vi "qmeter_calculation.vi"(1 "Range size":u16, 4 "Sample type":u16, 5 "Input voltage":dbl, 6 "stray capacitance":dbl, 7 "knob":dbl, 9 "phi":dbl, 10 "eta":dbl, 11 "trim":dbl) -> (2 "Cluster":cluster{"all rows":dbl[], "all rows":dbl[]})   [LabVIEW 2019]
uses:
  <vilib>/Utility/file.llb/Read Delimited Spreadsheet (DBL).vi
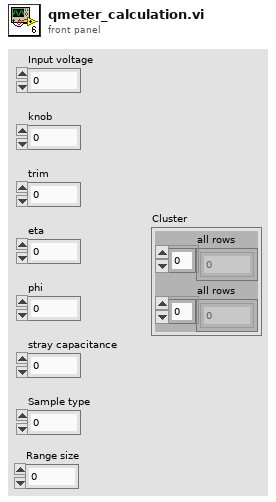
[diagram p1: front panel]
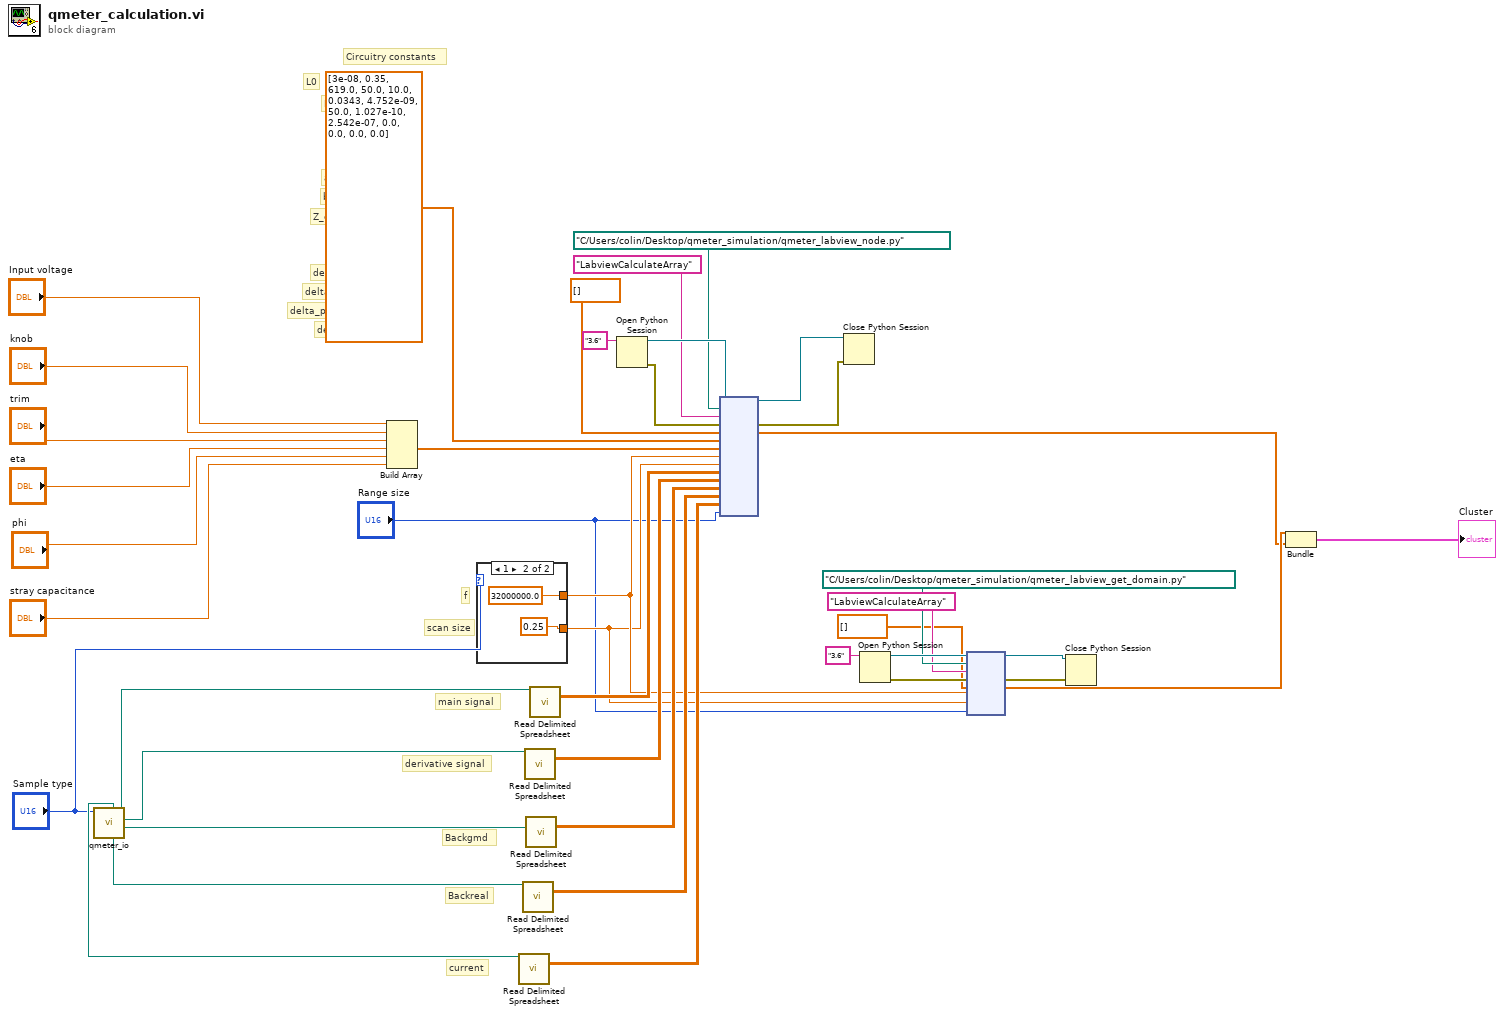
[diagram p0: block diagram]
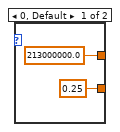
[diagram p2: hidden frame]
diagram:
  # "scan size"
  # "delta_phase"
  # "delta_l"
  # "delta_phi"
  # "delta_C"
  # "M"
  # "D"
  # "Z_cable"
  # "beta1"
  # "alpha"
  # "f"
  # "r"
  # "R1"
  # "R"
  # "Rcoil"
  # "L0"
  # "Circuitry constants"
  # "current"
  # "Backreal"
  # "Backgmd"
  # "derivative signal"
  # "main signal"
  n1 = call "qmeter_io.vi"("Sample type"="Sample type") -> ("file path (dialog if empty) 3"=w40:path, "file path (dialog if empty) 5"=w41:path, "file path (dialog if empty) 4"=w38:path, "file path (dialog if empty) 2"=w39:path, "file path (dialog if empty)"=w37:path)  [unwired: 6 in]
  n2 = Build Array("Input voltage", "knob", "trim", "eta", "phi", "stray capacitance") -> (w26:dbl[])
  n3 = case shown="1" "Sample type" {
    tunnel: [213000000.0 ("x+y") 32000000.0 ("x+y")] -> w8
    tunnel: [0.25 ("x+y") 0.25 ("x+y")] -> w7
    frame 0, Default {
    }
    frame 1 {
    }
  }
  n4 = call-poly <vilib>:"Read Delimited Spreadsheet.vi"("file path (dialog if empty)"=w37) -> ("all rows"=w27:dbl[][])  [unwired: 9 in, 5 out]
  n5 = call-poly <vilib>:"Read Delimited Spreadsheet.vi"("file path (dialog if empty)"=w39) -> ("all rows"=w28:dbl[][])  [unwired: 9 in, 5 out]
  n6 = call-poly <vilib>:"Read Delimited Spreadsheet.vi"("file path (dialog if empty)"=w41) -> ("all rows"=w30:dbl[][])  [unwired: 9 in, 5 out]
  n7 = call-poly <vilib>:"Read Delimited Spreadsheet.vi"("file path (dialog if empty)"=w40) -> ("all rows"=w29:dbl[][])  [unwired: 9 in, 5 out]
  n8 = call-poly <vilib>:"Read Delimited Spreadsheet.vi"("file path (dialog if empty)"=w38) -> ("all rows"=w31:dbl[][])  [unwired: 9 in, 5 out]
  n9 = Open Python Session(python version="3.6" ("Python version")) -> (session out=w22:refnum<k35>, error out=w20:errorcluster)  [unwired: 2 in]
  n10 = node(w22, path "C:/Users/colin/Desktop/qmeter_simulation/qmeter_labview_node.py" ("module path"), "LabviewCalculateArray" ("function name"), w20, dbl[] [], dbl[] [3e-08, 0.35, 619.0, 50.0, 10.0, 0.0343, 4.752e-09, 50.0, 1.027e-10, 2.542e-07, 0.0, 0.0, 0.0, 0.0], w26, w8, w7, w31, w30, w29, w28, w27, "Range size") -> (w21:refnum<k35>, w19:errorcluster, w2:dbl[])  [unwired: 10 in, 2 out]
  n11 = Close Python Session(session in=w21, error in=w19) -> ()  [unwired: 1 out]
  n12 = Open Python Session(python version="3.6" ("Python version")) -> (session out=w13:refnum<k35>, error out=w15:errorcluster)  [unwired: 2 in]
  n13 = node(w13, path "C:/Users/colin/Desktop/qmeter_simulation/qmeter_labview_get_domain.py" ("module path"), "LabviewCalculateArray" ("function name"), w15, dbl[] [], w8, w7, "Range size") -> (w5:refnum<k35>, w14:errorcluster, w3:dbl[])  [unwired: 3 in, 2 out]
  n14 = Close Python Session(session in=w5, error in=w14) -> ()  [unwired: 1 out]
  n15 = Bundle(w3, w2) -> (→"Cluster":cluster{dbl[], dbl[]})  [unwired: 1 in]
